vi "Camera_AcquireContinuousImage.vi"(0 "Stop (F)":bool, 1 "error in":errorcluster) -> (2 "Image Out":T1(plugin-control), 3 "Stopped":bool, 4 "error out":errorcluster)   [LabVIEW 2009, in "Camera.lvlib"]
uses:
  Camera.lvlib
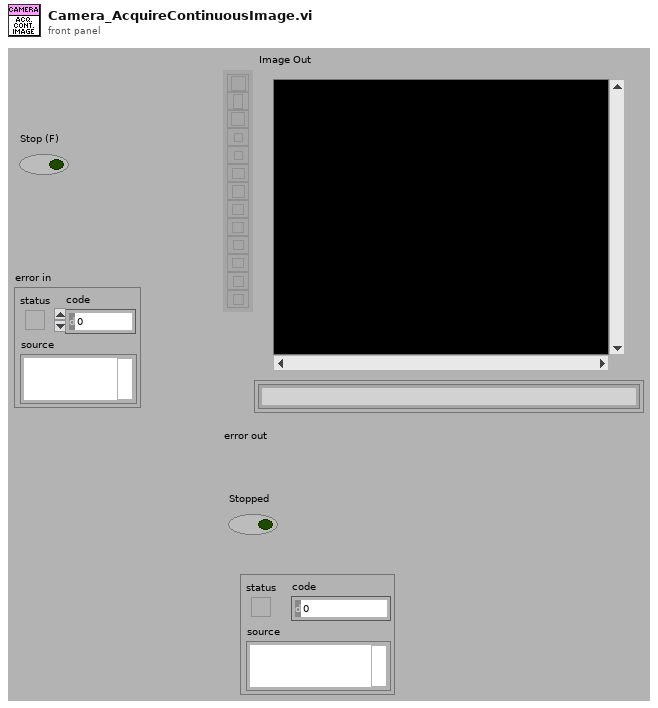
[diagram p1: front panel]
types:
  T1 = typedef "IMAQ Image.ctl" = refnum<image>
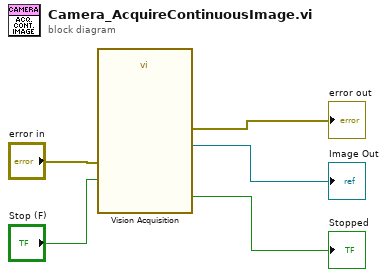
[diagram p0: block diagram]
diagram:
  n1 = call "Vision Acquisition"("Stop (F)"="Stop (F)", "error in"="error in") -> ("Image Out"=→"Image Out":T1, "Stopped"=→"Stopped":bool, "error out"=→"error out":errorcluster)  [unwired: 23 in]
